vi "Delay_Signal.vi"(1 "input":bool, 2 "Delay Signal (ms)":u32) -> (0 "output":bool)   [LabVIEW 2019]
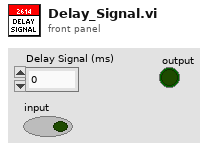
[diagram p1: front panel]
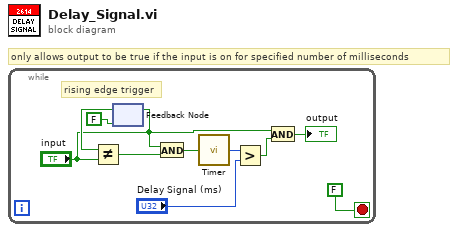
[diagram p0: block diagram]
diagram:
  # "only allows output to be true if the input is on for specified number of milliseconds"
  n1 = while {
    stop <- FALSE stop-if-true
    # "rising edge trigger"
    n2 = feedback-in #1("input") -> ()
    n3 = feedback #1(FALSE) -> (w4:bool)
    n4 = Not Equal?(x=w4, y="input") -> (x != y?=w3:bool)
    n5 = And(x="input", y=w3) -> (x .and. y?=w2:bool)
    n6 = call "Timer.vi"("Reset Timer"=w2) -> ("Time (ms)"=w7:u32)
    n7 = Greater?(x=w7, y="Delay Signal (ms)") -> (0:w9:bool)
    n8 = And(x="input", y=w9) -> (x .and. y?=→"output":bool)
  }
